vi "gaussian.vi"(2 "2-D Array of Real":dbl[][](array[numeric])) -> (5 "wx":dbl, 6 "x":dbl, 7 "y":dbl, 8 "xy":dbl, 9 "bkg":dbl, 10 "h":dbl)   [LabVIEW 2012]
panel:
  out "大小":i32[](array[numeric])
  out "1-D Array of Real":dbl[](array[numeric])
  out "exitflag":dbl
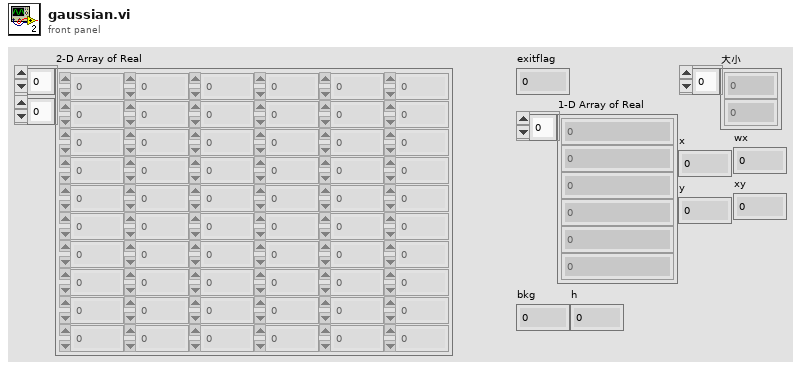
[diagram p1: front panel]
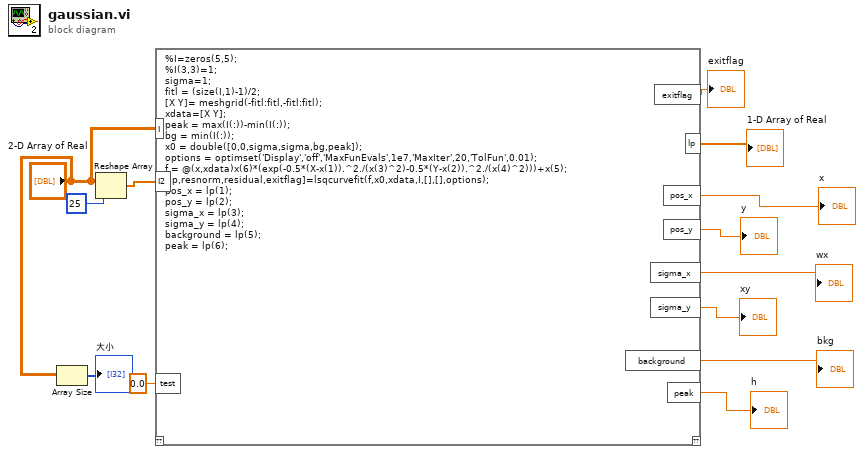
[diagram p0: block diagram]
diagram:
  n1 = Array Size(array="2-D Array of Real") -> (size(s)=→"大小":i32[])
  n2 = Reshape Array("2-D Array of Real", 25 ("维数大小")) -> (w10:dbl[])
  n3 = script code="%I=zeros(5,5);\n%I(3,3)=1;\nsigma=1;\nfitl = (size(I,1)-1)/2;\n[X Y]= meshgrid(-fitl:fitl,-fitl:fitl);\nxdata=[X Y];\npeak = max(I(:))-min(I(:));\nbg = min(I(:));\nx0 = double([0,0,sigma,sigma,bg,peak]);\noptions = optimset('Display','off','MaxFunEvals',1e7,'MaxIter',20,'TolFun',0.01);\nf = @(x,xdata)x(6)*(exp(-0.5*(X-x(1)).^2./(x(3)^2)-0.5*(Y-x(2)).^2./(x(4)^2)))+x(5);\n[lp,resnorm,residual,exitflag]=lsqcurvefit(f,x0,xdata,I,[],[],options);\npos_x = lp(1);\npos_y = lp(2);\nsigma_x = lp(3);\nsigma_y = lp(4);\nbackground = lp(5);\npeak = lp(6);"("test"=0.0 ("Real"), "I2"=w10, "I"="2-D Array of Real") -> ("exitflag"=→"exitflag":dbl, "lp"=→"1-D Array of Real":dbl[], "pos_x"=→"x":dbl, "pos_y"=→"y":dbl, "sigma_x"=→"wx":dbl, "sigma_y"=→"xy":dbl, "background"=→"bkg":dbl, "peak"=→"h":dbl)  [unwired: 1 in, 1 out]
